vi "Generate PriceData Waveform.vi"(9 "PriceData_RealTime_Backup":variant, 10 "Max Forecast Length":i32, 11 "Generic Optimization in":refnum<class "Generic Optimization.lvclass">) -> (1 "Waveform":waveform(dbl), 2 "PriceData_RealTime":T1, 3 "dup Generic Optimization out":refnum<class "Generic Optimization.lvclass">)   [LabVIEW 2018, in "Generic Optimization Actor.lvlib" / "Generic Optimization.lvclass"]
uses:
  Generic Optimization.lvclass
  <vilib>/ORNL/CSEISMIC DDS/CSEISMIC DDS Base/Data Types/PriceData_RealTime.ctl
  <vilib>/ORNL/CSEISMIC DDS/CSEISMIC DDS Base/Data Types/Controls/DeviceID.ctl
  C:/Users/Administrator/Desktop/2018LabVIEW EMS/EMS Generic Actor/EMS Generic/EMS Generic.lvclass
  <vilib>/ORNL/CSEISMIC DDS/CSEISMIC DDS Base/CSEISMIC DDS.lvclass
  EMS Generic Actor/EMS Generic/EMS Generic.lvclass
  Utilities/Status Messaging.llb/Status Messaging.lvlib
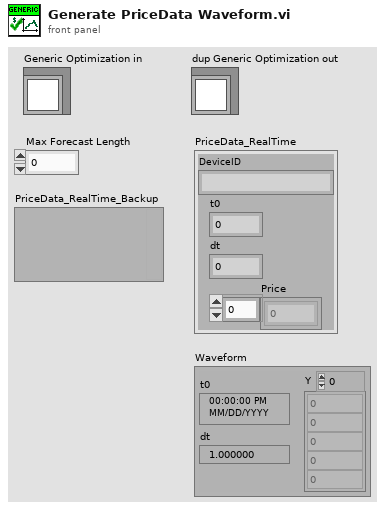
[diagram p1: front panel]
types:
  T1 = typedef "CSEISMIC DDS.lvlib/CSEISMIC DDS.lvclass/PriceData_RealTime.ctl" = cluster{"DeviceID":T2, "t0":dbl, "dt":dbl, "Price":dbl[]}
  T2 = typedef "CSEISMIC DDS.lvlib/CSEISMIC DDS.lvclass/DeviceID.ctl" = string
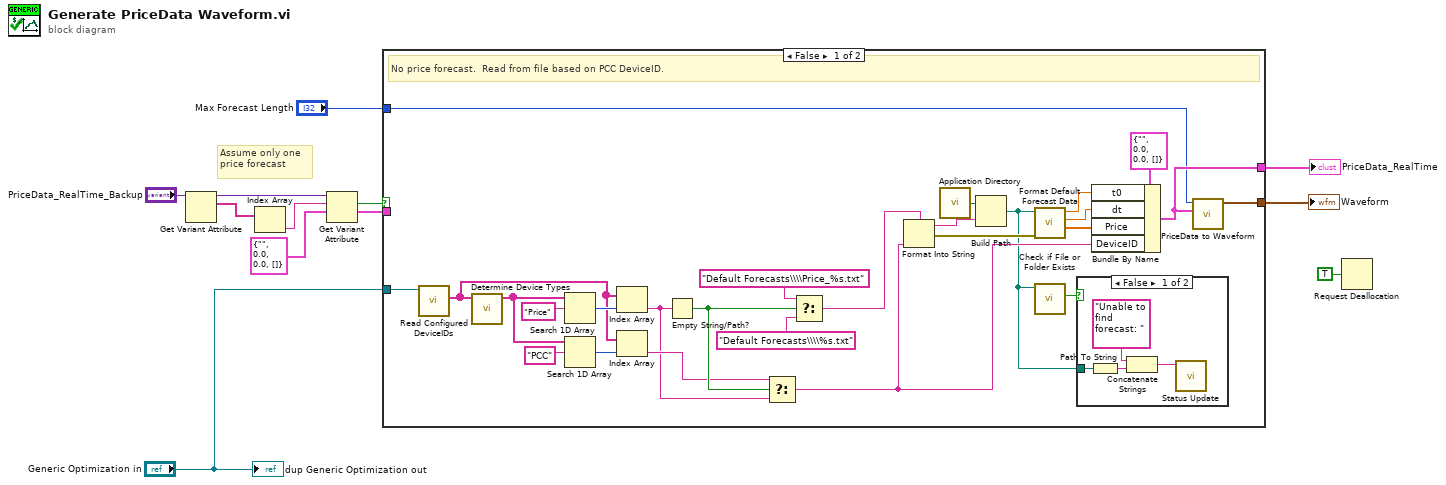
[diagram p0: block diagram]
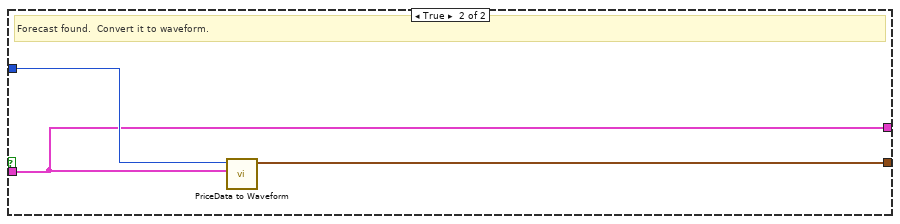
[diagram p3: hidden frame]
diagram:
  # "Assume only one price forecast"
  n1 = Get Variant Attribute(Variant="PriceData_RealTime_Backup") -> (duplicate Variant=w6:variant, names=w5:string[])  [unwired: 3 in, 2 out]
  n2 = Index Array(array=w5) -> (element=w7:string)  [unwired: 1 in]
  n3 = Get Variant Attribute(Variant=w6, name=w7, default value (empty Variant)=T1 {"DeviceID"="", "t0"=0.0, "dt"=0.0, "Price"=[]} ("PriceData_RealTime")) -> (found=w4:bool, value=w11:T1)  [unwired: 1 in, 2 out]
  n4 = case shown="False" w4 {
    tunnel: w11 -> [_ w43]
    tunnel: "Max Forecast Length" -> [w29 w45]
    tunnel: [w30 w44] -> w9
    tunnel: [w31 w43] -> w3
    tunnel: "Generic Optimization in" -> [w28 _]
    frame False {
      # "No price forecast.  Read from file based on PCC DeviceID."
      n5 = call "Read Configured DeviceIDs.vi"("EMS Generic in"=w28) -> ("DeviceIDs"=w22:T2[])  [unwired: 8 in, 2 out]
      n6 = call "Determine Device Types.vi"("DeviceIDs"=w22) -> ("Device Classes"=w23:string[])  [unwired: 9 in]
      n7 = Search 1D Array(1D array=w23, element="Price") -> (index of element=w26:i32)  [unwired: 1 in]
      n8 = Search 1D Array(1D array=w23, element="PCC") -> (index of element=w24:i32)  [unwired: 1 in]
      n9 = Index Array(array=w22, index=w26) -> (element=w17:T2)
      n10 = Index Array(array=w22, index=w24) -> (element=w18:T2)
      n11 = Empty String/Path?(string/path=w17) -> (empty?=w19:bool)
      n12 = Select(t=w18, s=w19, f=w17) -> (s? t:f=w16:T2)
      n13 = Select(t="Default Forecasts\\\\Price_%s.txt" ("format string"), s=w19, f="Default Forecasts\\\\%s.txt" ("format string")) -> (s? t:f=w14:string)
      n14 = Format Into String(format string=w14, w16) -> (resulting string=w37:string, error out=w36:errorcluster)  [unwired: 2 in]
      n15 = call <vilib>:"Application Directory.vi"() -> ("Application Directory"=w38:path)
      n16 = Build Path(base path=w38, name or relative path=w37) -> (appended path=w13:path)
      n17 = call "Format Default Forecast Data.vi"("error in"=w36, "file path"=w13) -> ("Data"=w32:dbl[], "dt (sec)"=w33:dbl, "t0 (sec)"=w34:dbl)  [unwired: 6 in, 1 out]
      n18 = call <vilib>:"Check if File or Folder Exists.vi"("path"=w13) -> ("file or folder exists?"=w15:bool)  [unwired: 8 in, 2 out]
      n19 = case shown="False" w15 {
        tunnel: w13 -> [w39 _]
        frame False {
          n20 = Path To String(path=w39) -> (string=w40:string)
          n21 = Concatenate Strings("Unable to find forecast: " ("string"), w40) -> (w41:string)
          n22 = call "Status Update.vi"("Status Update"=w41) -> ()  [unwired: 9 in, 2 out]
        }
        frame True {
        }
      }
      n23 = Bundle By Name(cluster=T1 {"DeviceID"="", "t0"=0.0, "dt"=0.0, "Price"=[]} ("PriceData_RealTime"), "t0"=w34, "dt"=w33, "Price"=w32, "DeviceID"=w16) -> (w31:T1)
      n24 = call "PriceData to Waveform.vi"("PriceData_RealTime"=w31, "Max Forecast Length"=w29) -> ("Waveform"=w30:waveform(dbl))  [unwired: 9 in]
    }
    frame True {
      # "Forecast found.  Convert it to waveform."
      n25 = call "PriceData to Waveform.vi"("PriceData_RealTime"=w43, "Max Forecast Length"=w45) -> ("Waveform"=w44:waveform(dbl))  [unwired: 9 in]
    }
  }
  "PriceData_RealTime" <- w3
  "Waveform" <- w9
  n26 = Request Deallocation(TRUE ("flag")) -> ()
  "dup Generic Optimization out" <- "Generic Optimization in"
